vi "电源管理UI.vi"() -> ()   [LabVIEW 2016, in "PLC.lvlib"]
uses:
  PLC.lvlib
  <vilib>/Utility/miscctls.llb/LVPointTypeDef.ctl
  API/CodCr/CodCr.lvlib
panel:
  out "CODCr空闲时间":dbl caption="空闲时间:"
  out "总磷总氮空闲时间":dbl caption="空闲时间:"
  out "营养盐空闲时间":dbl caption="空闲时间:"
  out "CODMn空闲时间":dbl caption="空闲时间:"
  out "多参数空闲时间":dbl caption="空闲时间:"
  in  "CODCr电源":bool
  in  "总磷总氮电源":bool
  in  "营养盐电源":bool
  in  "CODMn电源":bool
  in  "多参数电源":bool
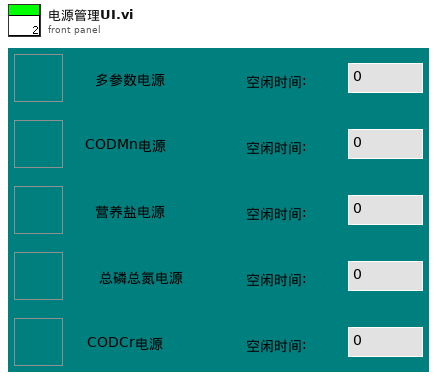
[diagram p1: front panel]
types:
  T1 = typedef "LVPointTypeDef.ctl" = cluster{"Horizontal":i16, "Vertical":i16}
  T2 = enum16{"空闲", "水样测试", "标样核查", "零点核查", "跨度核查", "空白测试", "平行样测试", "加标回收", "空白校准", "标样校准", "初始化（清洗）"}
  T3 = cluster{"系统时间":timestamp, "工作状态":u16, "测量模式":u16, "告警代码":enum16{"无告警", "缺试剂告警", "缺水样告警", "缺蒸馏水告警", "缺标液告警", "仪表漏液告警", "标定异常告警", "超量程告警", "加热异常", "低试剂预警", "超上限告警", "超下限告警", "仪表内部其他异常", "滴定异常告警", "电极异常告警", "量程切换告警", "参数设置告警", "PH电极电位异常", "电导率电极异常", "浊度光度异常", "溶解氧电极异常", "溶解氧光强异常", "温度异常告警", "PH异常告警", "溶解氧异常告警", "电导率异常告警", "浊度异常告警", "叶绿素异常告警", "藻密度异常告警", "蓝绿藻异常告警", "ORP异常告警", "氨氮异常告警", "清洁刷异常告警", "SD卡异常告警", "蓝牙异常告警", "Wifi异常告警", "流程异常告警"}, "故障代码":enum16{"无故障", "电机故障", "温度故障", "通讯故障", "滴定故障"}, "日志代码":u16, "软件版本":string}
  T4 = cluster{"系统时间":timestamp, "工作状态":enum16{"空闲", "水样测试", "标样核查", "零点核查", "跨度核查", "空白测试", "平行样测试", "加标回收", "空白校准", "标样校准", "初始化（清洗）"}, "测量模式":enum16{"待机", "连续模式", "周期模式", "定点模式", "受控模式", "手动模式"}, "告警代码":enum16{"无告警", "缺试剂告警", "缺水样告警", "缺蒸馏水告警", "缺标液告警", "仪表漏液告警", "标定异常告警", "超量程告警", "加热异常", "低试剂预警", "超上限告警", "超下限告警", "仪表内部其他异常", "滴定异常告警", "电极异常告警", "量程切换告警", "参数设置告警", "PH电极电位异常", "电导率电极异常", "浊度光度异常", "溶解氧电极异常", "溶解氧光强异常", "温度异常告警", "PH异常告警", "溶解氧异常告警", "电导率异常告警", "浊度异常告警", "叶绿素异常告警", "藻密度异常告警", "蓝绿藻异常告警", "ORP异常告警", "氨氮异常告警", "清洁刷异常告警", "SD卡异常告警", "蓝牙异常告警", "Wifi异常告警", "流程异常告警"}, "故障代码":enum16{"无故障", "电机故障", "温度故障", "通讯故障", "滴定故障"}, "日志代码":u16, "软件版本":u16, "F0":sgl, "F1":sgl, "F2":sgl, "F3":sgl, "T":sgl, "H":sgl, "id":u16, "flowid":u16, "量程":u16}
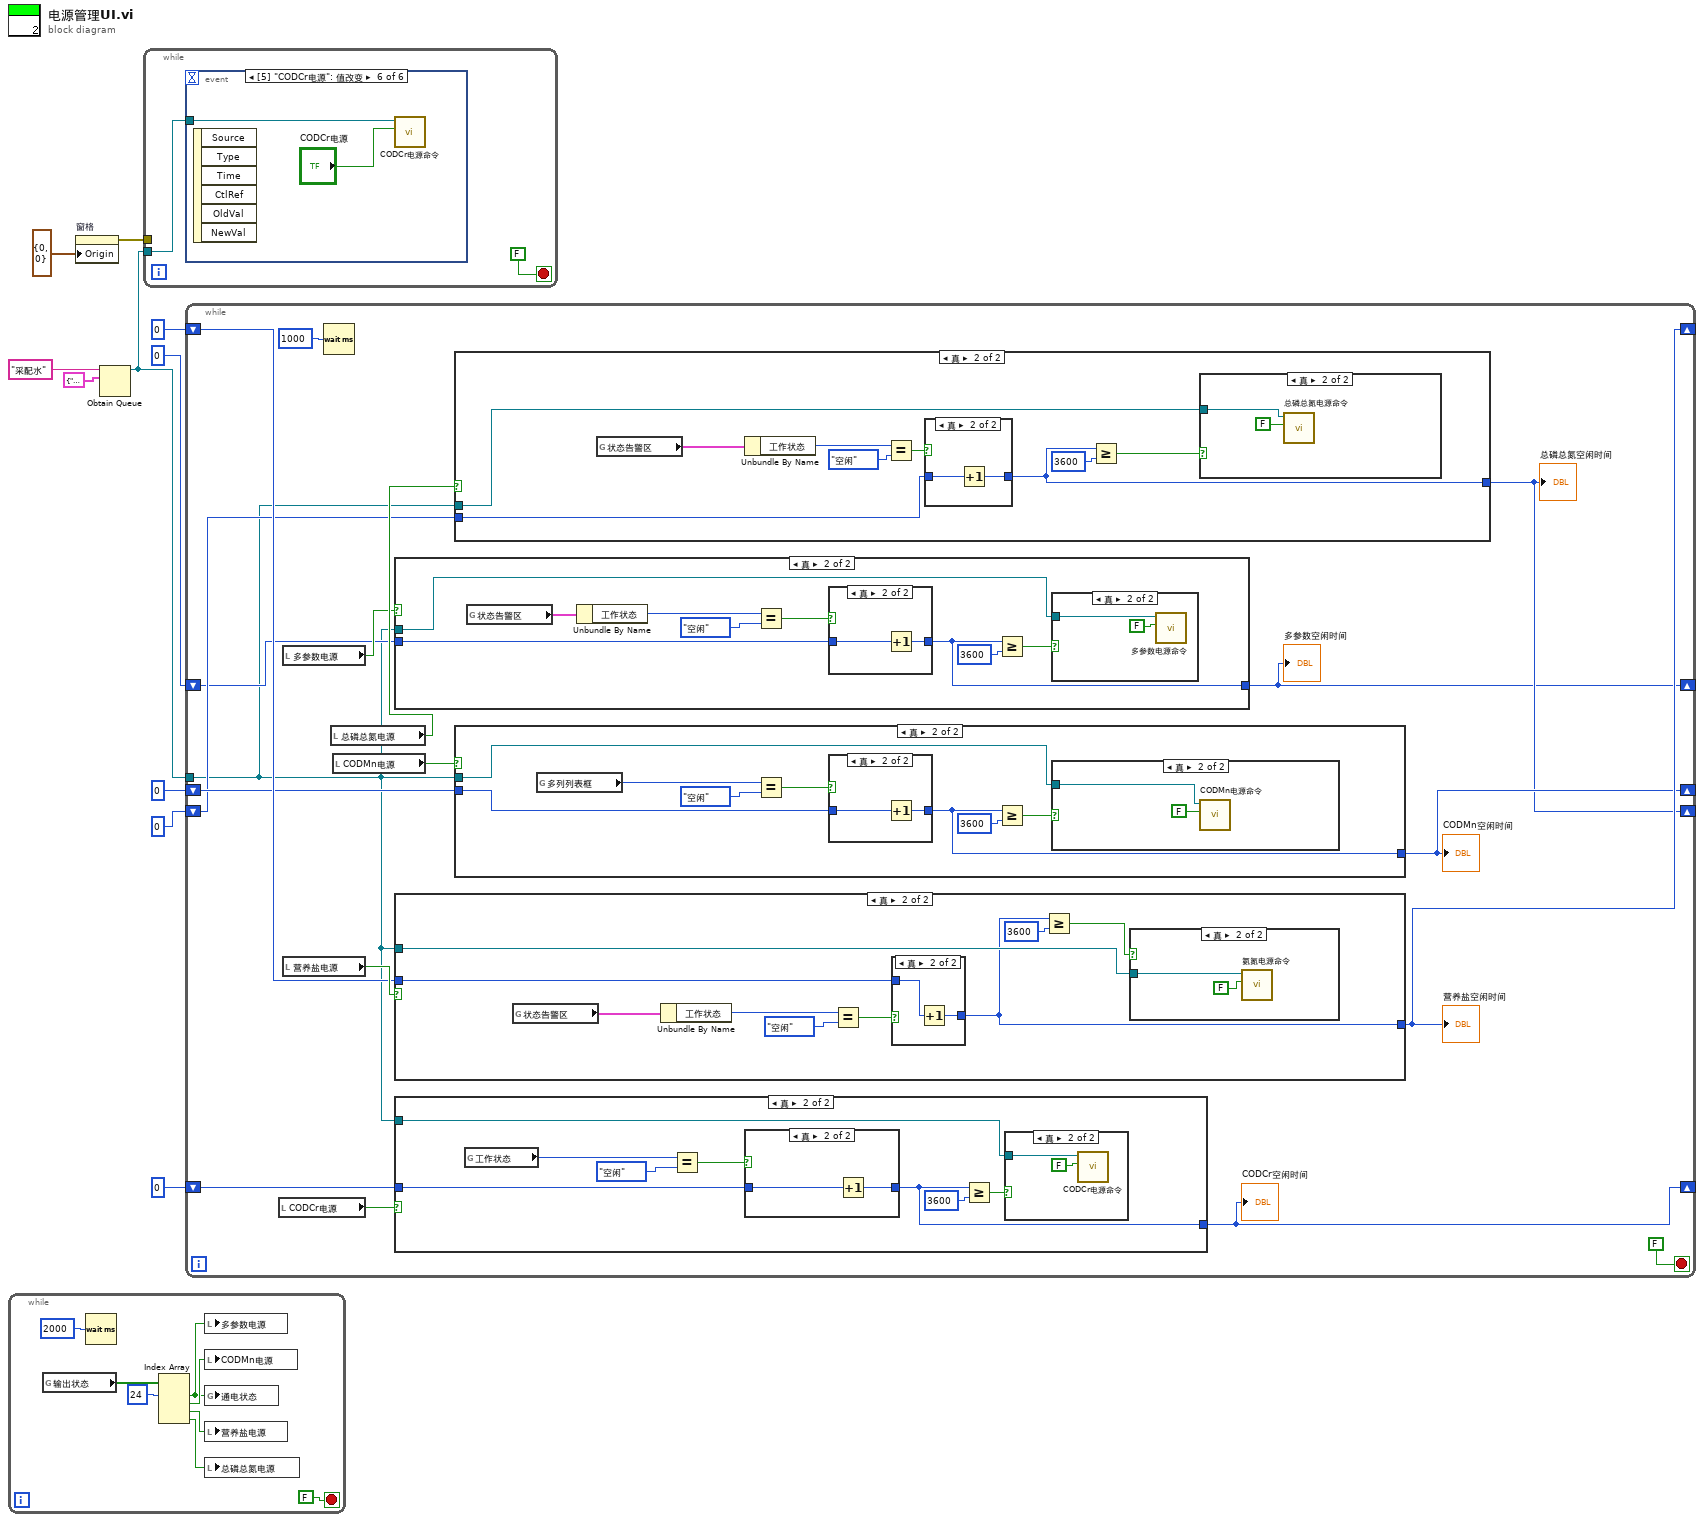
[diagram p0: block diagram]
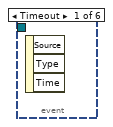
[diagram p17: hidden frame]
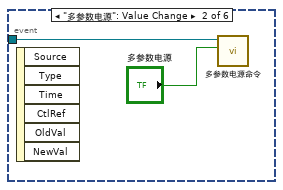
[diagram p18: hidden frame]
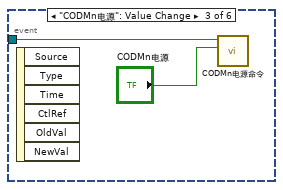
[diagram p19: hidden frame]
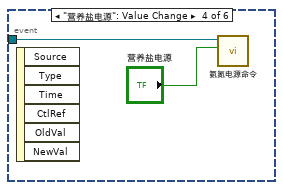
[diagram p20: hidden frame]
diagram:
  n1 = while {
    stop <- FALSE stop-if-true
    n2 = global read "采配水全局变量.vi" "输出状态"() -> (w16:bool[])
    n3 = Wait (ms)(milliseconds to wait=u32 2000 ("等待时间（毫秒）")) -> ()  [unwired: 1 out]
    n4 = Index Array(array=w16, index #1=24 ("索引")) -> (element #1=w11:bool, element #2=w14:bool, element #3=w13:bool, element #4=w12:bool)  [unwired: 3 in]
    n5 = local write "多参数电源"(w11) -> ()
    n6 = local write "CODMn电源"(w14) -> ()
    n7 = global write "多参数全局变量.vi" "通电状态"(w11) -> ()
    n8 = local write "营养盐电源"(w13) -> ()
    n9 = local write "总磷总氮电源"(w12) -> ()
  }
  n10 = property on="窗格" class="Pane"("Origin"=T1 {"Horizontal"=0, "Vertical"=0} ("原点")) -> (error out=w7:errorcluster)  [unwired: 2 in, 1 out]
  n11 = Obtain Queue(name (unnamed)="采配水" ("名称（未命名）"), element data type=cluster{"命令":string, "数据":variant} {"命令"="", "数据"=variant}) -> (queue out=w6:refnum<queue>)  [unwired: 3 in, 2 out]
  n12 = while {
    tunnel: w6 -> [w19]
    tunnel: w7 -> [_]
    stop <- FALSE stop-if-true
    n13 = event shown="[5] \"CODCr电源\": 值改变" {
      selector: _ -> [_ _ _ _ _ _]
      dyn-events: _ -> [_ _ _ _ _ _]
      timeout: _ -> [_ _ _ _ _ _]
      tunnel: w19 -> [_ w22 w24 w26 w28 w30]
      event Timeout {
        n14 = event-data() -> ()  [unwired: 1 in, 3 out]
      }
      event "多参数电源": Value Change {
        n15 = event-data() -> ()  [unwired: 1 in, 6 out]
        n16 = call "多参数电源命令.vi"("通电/断电"="多参数电源", "队列"=w22) -> ()  [unwired: 9 in, 1 out]
      }
      event "CODMn电源": Value Change {
        n17 = event-data() -> ()  [unwired: 1 in, 6 out]
        n18 = call "CODMn电源命令.vi"("通电/断电"="CODMn电源", "队列"=w24) -> ()  [unwired: 9 in, 1 out]
      }
      event "营养盐电源": Value Change {
        n19 = event-data() -> ()  [unwired: 1 in, 6 out]
        n20 = call "氨氮电源命令.vi"("通电/断电"="营养盐电源", "队列"=w26) -> ()  [unwired: 9 in, 1 out]
      }
      event "总磷总氮电源": Value Change {
        n21 = event-data() -> ()  [unwired: 1 in, 6 out]
        n22 = call "总磷总氮电源命令.vi"("通电/断电"="总磷总氮电源", "队列"=w28) -> ()  [unwired: 9 in, 1 out]
      }
      event "CODCr电源": Value Change {
        n23 = event-data() -> ()  [unwired: 1 in, 6 out]
        n24 = call "CODCr电源命令.vi"("通电/断电"="CODCr电源", "队列"=w30) -> ()  [unwired: 9 in, 1 out]
      }
    }
  }
  n25 = while {
    tunnel: w6 -> [w37]
    shift-right: [w35] -> _
    shift-left: u32 0 ("等待时间（毫秒）") -> [w45]
    shift-right: [w34] -> _
    shift-left: u32 0 ("等待时间（毫秒）") -> [w43]
    shift-right: [w32] -> _
    shift-left: u32 0 ("等待时间（毫秒）") -> [w39]
    shift-right: [w33] -> _
    shift-left: u32 0 ("等待时间（毫秒）") -> [w40]
    shift-right: [w31] -> _
    shift-left: u32 0 ("等待时间（毫秒）") -> [w38]
    stop <- FALSE stop-if-true
    n26 = local read "CODCr电源"() -> (w36:bool)
    n27 = local read "多参数电源"() -> (w41:bool)
    n28 = local read "营养盐电源"() -> (w46:bool)
    n29 = Wait (ms)(milliseconds to wait=u32 1000 ("等待时间（毫秒）")) -> ()  [unwired: 1 out]
    n30 = local read "总磷总氮电源"() -> (w42:bool)
    n31 = local read "CODMn电源"() -> (w44:bool)
    n32 = case shown="真" w41 {
      tunnel: w39 -> [_ w69]
      tunnel: [_ w65] -> w32
      tunnel: w37 -> [_ w66]
      frame False {
      }
      frame True {
        n33 = global read "多参数全局变量.vi" "状态告警区"() -> (w62:T3)
        n34 = Unbundle By Name(w62) -> ("工作状态"=w61:u16)
        n35 = Equal?(x=w61, y=T2."空闲" ("工作状态")) -> (x = y?=w67:bool)
        n36 = case shown="真" w67 {
          tunnel: w69 -> [_ w73]
          tunnel: [_ w72] -> w65
          frame False {
          }
          frame True {
            n37 = Increment(x=w73) -> (x+1=w72:u32)
          }
        }
        n38 = Greater Or Equal?(x=w65, y=u32 3600) -> (x >= y?=w63:bool)
        n39 = case shown="真" w63 {
          tunnel: w66 -> [_ w71]
          frame False {
          }
          frame True {
            n40 = call "多参数电源命令.vi"("通电/断电"=FALSE, "队列"=w71) -> ()  [unwired: 9 in, 1 out]
          }
        }
      }
    }
    "多参数空闲时间" <- w32
    n41 = case shown="真" w46 {
      tunnel: w45 -> [_ w107]
      tunnel: [_ w101] -> w35
      tunnel: w37 -> [_ w102]
      frame False {
      }
      frame True {
        n42 = global read "VAR总磷氨氮全局变量.vi" "状态告警区"() -> (w106:T4)
        n43 = Unbundle By Name(w106) -> ("工作状态"=w105:T2)
        n44 = Equal?(x=w105, y=T2."空闲" ("工作状态")) -> (x = y?=w103:bool)
        n45 = case shown="真" w103 {
          tunnel: w107 -> [_ w111]
          tunnel: [_ w110] -> w101
          frame False {
          }
          frame True {
            n46 = Increment(x=w111) -> (x+1=w110:u32)
          }
        }
        n47 = Greater Or Equal?(x=w101, y=u32 3600) -> (x >= y?=w99:bool)
        n48 = case shown="真" w99 {
          tunnel: w102 -> [_ w109]
          frame False {
          }
          frame True {
            n49 = call "氨氮电源命令.vi"("通电/断电"=FALSE, "队列"=w109) -> ()  [unwired: 9 in, 1 out]
          }
        }
      }
    }
    "营养盐空闲时间" <- w35
    n50 = case shown="真" w36 {
      tunnel: w38 -> [_ w56]
      tunnel: [_ w52] -> w31
      tunnel: w37 -> [_ w53]
      frame False {
      }
      frame True {
        n51 = global read "CODcr全局变量.vi" "工作状态"() -> (w49:T2)
        n52 = Equal?(x=w49, y=T2."空闲" ("工作状态")) -> (x = y?=w54:bool)
        n53 = case shown="真" w54 {
          tunnel: w56 -> [_ w60]
          tunnel: [_ w59] -> w52
          frame False {
          }
          frame True {
            n54 = Increment(x=w60) -> (x+1=w59:u32)
          }
        }
        n55 = Greater Or Equal?(x=w52, y=u32 3600) -> (x >= y?=w50:bool)
        n56 = case shown="真" w50 {
          tunnel: w53 -> [_ w58]
          frame False {
          }
          frame True {
            n57 = call "CODCr电源命令.vi"("通电/断电"=FALSE, "队列"=w58) -> ()  [unwired: 9 in, 1 out]
          }
        }
      }
    }
    "CODCr空闲时间" <- w31
    n58 = case shown="真" w42 {
      tunnel: w40 -> [_ w82]
      tunnel: [_ w78] -> w33
      tunnel: w37 -> [_ w79]
      frame False {
      }
      frame True {
        n59 = global read "VAR总磷氨氮全局变量.vi" "状态告警区"() -> (w75:T4)
        n60 = Unbundle By Name(w75) -> ("工作状态"=w74:T2)
        n61 = Equal?(x=w74, y=T2."空闲" ("工作状态")) -> (x = y?=w80:bool)
        n62 = case shown="真" w80 {
          tunnel: w82 -> [_ w86]
          tunnel: [_ w85] -> w78
          frame False {
          }
          frame True {
            n63 = Increment(x=w86) -> (x+1=w85:u32)
          }
        }
        n64 = Greater Or Equal?(x=w78, y=u32 3600) -> (x >= y?=w76:bool)
        n65 = case shown="真" w76 {
          tunnel: w79 -> [_ w84]
          frame False {
          }
          frame True {
            n66 = call "总磷总氮电源命令.vi"("通电/断电"=FALSE, "队列"=w84) -> ()  [unwired: 9 in, 1 out]
          }
        }
      }
    }
    "总磷总氮空闲时间" <- w33
    n67 = case shown="真" w44 {
      tunnel: w43 -> [_ w94]
      tunnel: [_ w90] -> w34
      tunnel: w37 -> [_ w91]
      frame False {
      }
      frame True {
        n68 = global read "运行时序全局变量.vi" "多列列表框"() -> (w87:i32)
        n69 = Equal?(x=w87, y=T2."空闲" ("工作状态")) -> (x = y?=w92:bool)
        n70 = case shown="真" w92 {
          tunnel: w94 -> [_ w98]
          tunnel: [_ w97] -> w90
          frame False {
          }
          frame True {
            n71 = Increment(x=w98) -> (x+1=w97:u32)
          }
        }
        n72 = Greater Or Equal?(x=w90, y=u32 3600) -> (x >= y?=w88:bool)
        n73 = case shown="真" w88 {
          tunnel: w91 -> [_ w96]
          frame False {
          }
          frame True {
            n74 = call "CODMn电源命令.vi"("通电/断电"=FALSE, "队列"=w96) -> ()  [unwired: 9 in, 1 out]
          }
        }
      }
    }
    "CODMn空闲时间" <- w34
  }
